vi "LDA_Beam_Alignment.vi"() -> ()   [LabVIEW 2021]
uses:
  Anemometry Sub Vis/Controls/Beam_Type.ctl
  Anemometry Sub Vis/Controls/Fixed Axis.ctl
  Anemometry Sub Vis/Gen Trav/Traverse_cluster.ctl
  Anemometry Sub Vis/Gen Trav/Spacing.ctl
  Anemometry Sub Vis/Controls/Multi_run_mode.ctl
  Anemometry Sub Vis/Controls/User_Specific_mode.ctl
  Anemometry Sub Vis/Controls/Tunnel_Coordinates.ctl
  Anemometry Sub Vis/Controls/Post_Process.ctl
  Anemometry Sub Vis/Gen Trav/Trav_mode.ctl
  Anemometry Sub Vis/Globals/Trav_pos_global.vi
  Anemometry Sub Vis/Globals/Meas_global.vi
panel:
  out "String":string
  in  "Peak up":bool[](array[boolean])
  out "Fixed Axis":T1
  out "Beam Names":string[](array[string])
  in  "Mode":T2(ring)
  out "Values Out":dbl[][](array[numeric])
  out "Message":string
  in  "Go Back":bool
  in  "OK":bool
  in  "stop":bool
  in  "Working On":T3 items=["532 Unshifted", "532 shifted", "561 Unshfited", "561 Shfited", "553 Unshfited", "553 Shfited"]
  # "X                 Y              Z           Power mW"
  # "X                 Y              Z"
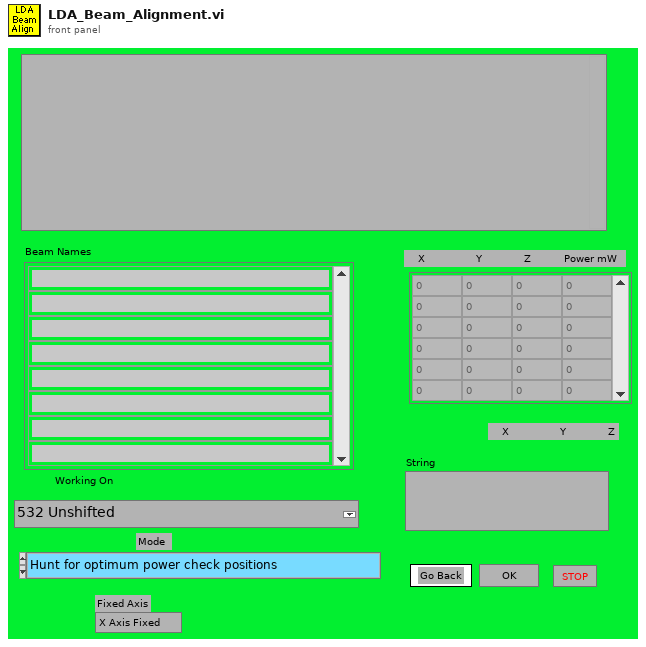
[diagram p1: front panel]
types:
  T1 = typedef "Fixed Axis.ctl" = enum16{"X Axis Fixed", "Y Axis Fixed", "Z Axis Fixed"}
  T2 = enum16{"Hunt for optimum power check positions", "Check Beam powers now", "Peak up beam power using manipulators"}
  T3 = typedef "Beam_Type.ctl" = u16
  T4 = typedef "Traverse_cluster.ctl" = cluster{"Start X":sgl, "Start Y":sgl, "Start Z":sgl, "End X":sgl, "End Y":sgl, "End Z":sgl, "nPoints":i32, "Spacing":T5, "Filename":path, "Tunnel Speed":dbl, "Averaging time (mins)":dbl, "Extra Commands":string, "Carrier_1 Q (l/min)":dbl, "Carrier_2 Q (l/min)":dbl, "Trace Gas Concentration (%)":dbl, "Specific Arguments":string, "Comments":string, "Row No":i32, "Row Type Selector":T6, "EstCompl":string, "Row Duration (mins)":dbl, "nValidPoints":i32, "Meas Setup File":string}
  T5 = typedef "Spacing.ctl" = enum16{"Linear", "Log", "Gauss", "Specified", "N/A"}
  T6 = typedef "Multi_run_mode.ctl" = enum16{"Move Traverse Only", "Set Tunnel Speed Only", "Set Source Only", "Set Measurement Conditions", "Single Measurement", "Vertical Profile", "Lateral Profile", "Longitudinal Profile", "Multi-Axis Profile", "Explore Volume", "Auto Calibrate", "Meas Fast FID Bkgnd", "Check Beam Power", "Scanning Valve Measurement", "Run VI Named:", "Set ADAM Ch", "Wait (minutes)", "Send Message", "Synchronize With:", "Fall Back to this Row", "Turn Off Row Repeating", "Traverse 3D Volume", "Blank Row", "Jump to Fall Back Row"}
  T7 = cluster{"Position":dbl[], "Traverse Name":string}[][]
  T8 = typedef "Tunnel_Coordinates.ctl" = enum16{"Work in Tunnel Coordinates", "Work in Model Coordinates"}
  T9 = typedef "User_Specific_mode.ctl" = enum16{"Check VI only", "Run VI"}
  T10 = typedef "Post_Process.ctl" = enum16{"Take New Data", "Post Process Raw Data File"}
  T11 = typedef "Trav_mode.ctl" = enum16{"Move traverse", "Read traverse position", "Teach Position"}
  T12 = cluster{"Position":dbl[], "Traverse Name":string}[]
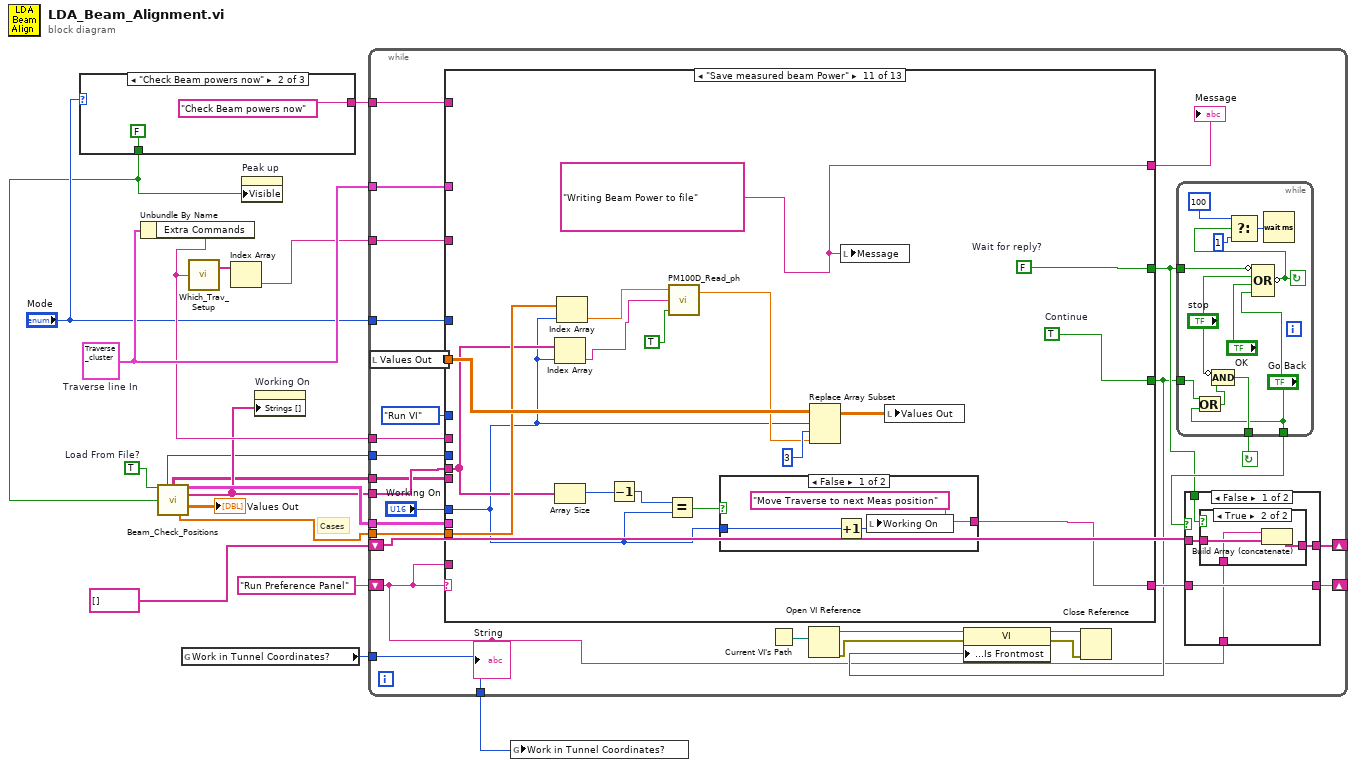
[diagram p0: block diagram]
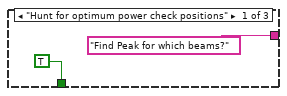
[diagram p2: hidden frame]
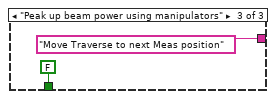
[diagram p3: hidden frame]
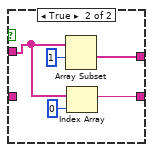
[diagram p5: hidden frame]
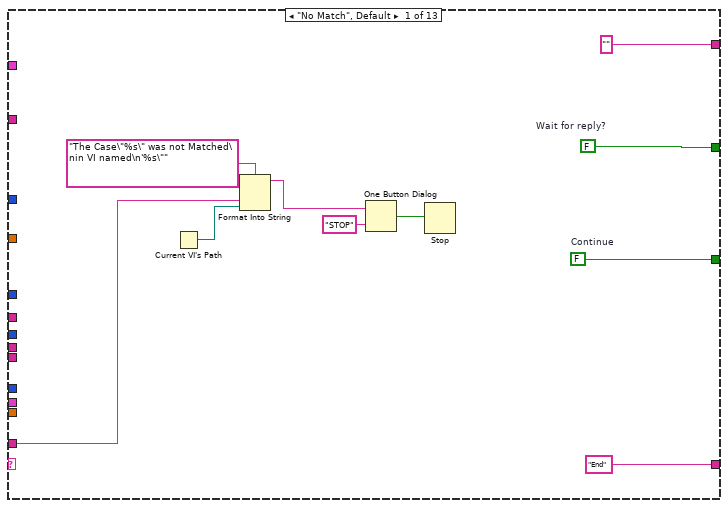
[diagram p6: hidden frame]
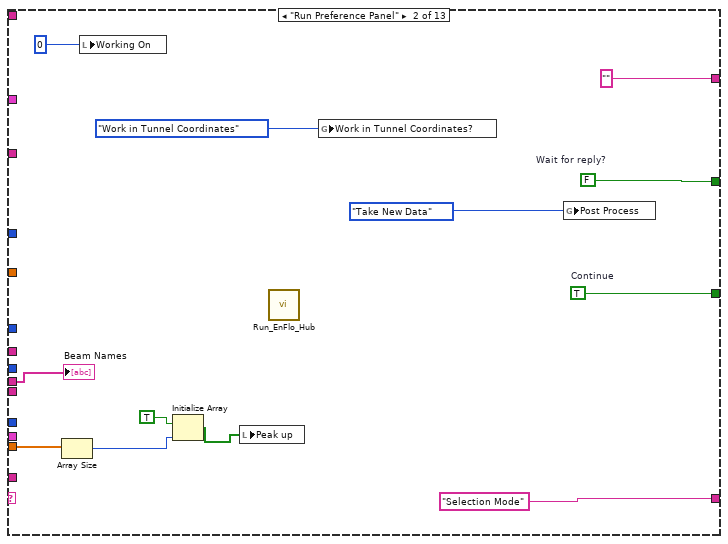
[diagram p7: hidden frame]
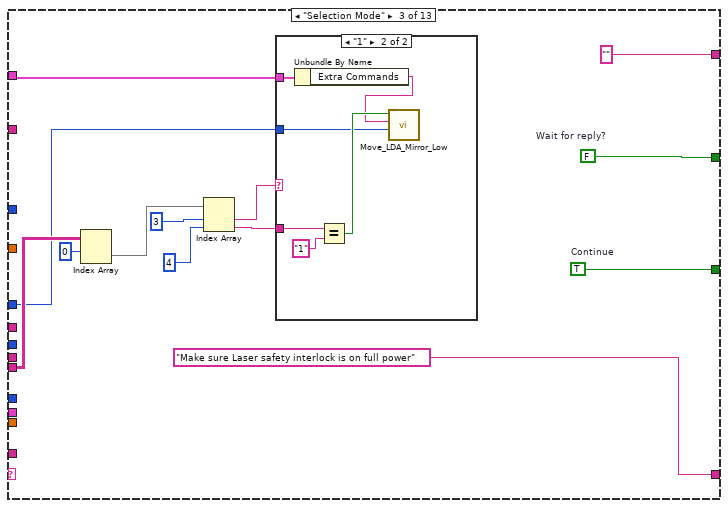
[diagram p8: hidden frame]
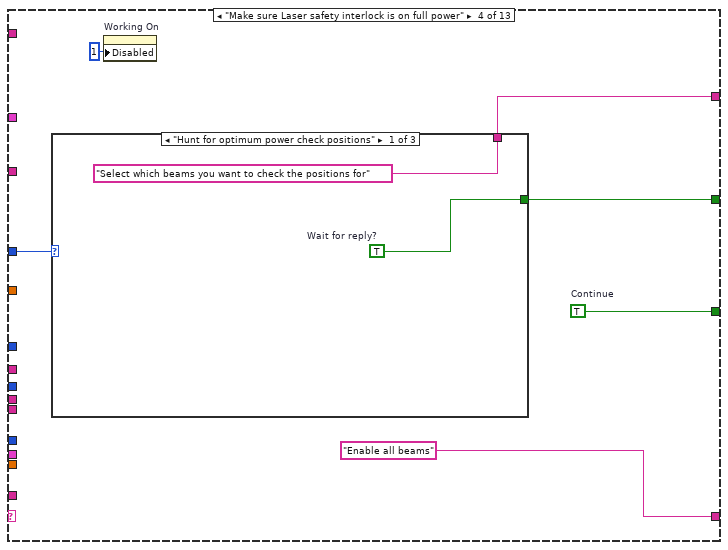
[diagram p10: hidden frame]
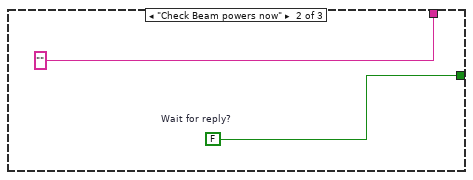
[diagram p11: hidden frame]
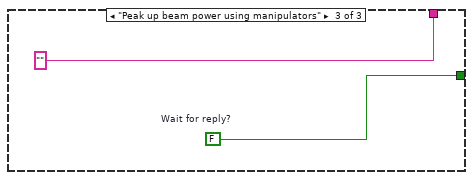
[diagram p12: hidden frame]
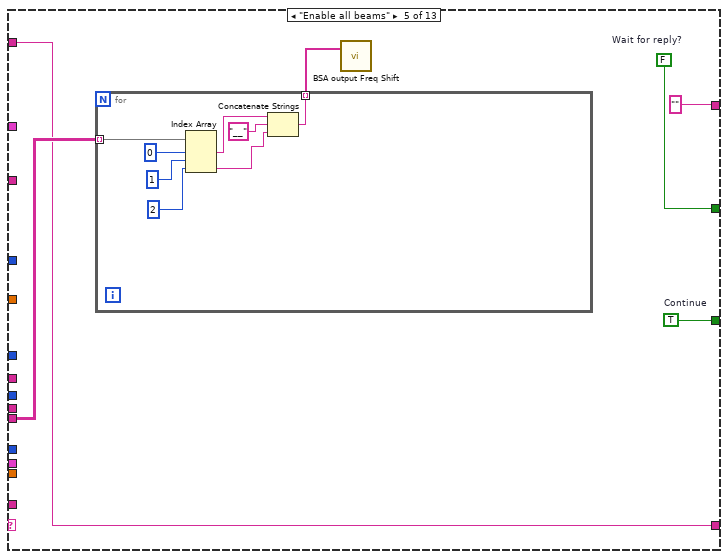
[diagram p13: hidden frame]
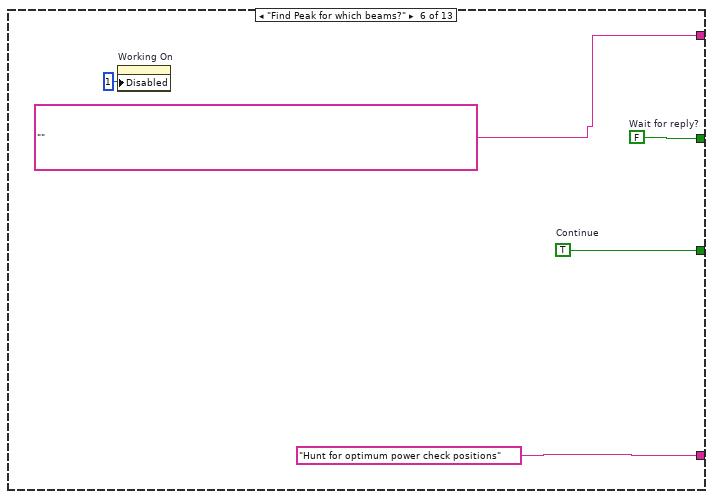
[diagram p14: hidden frame]
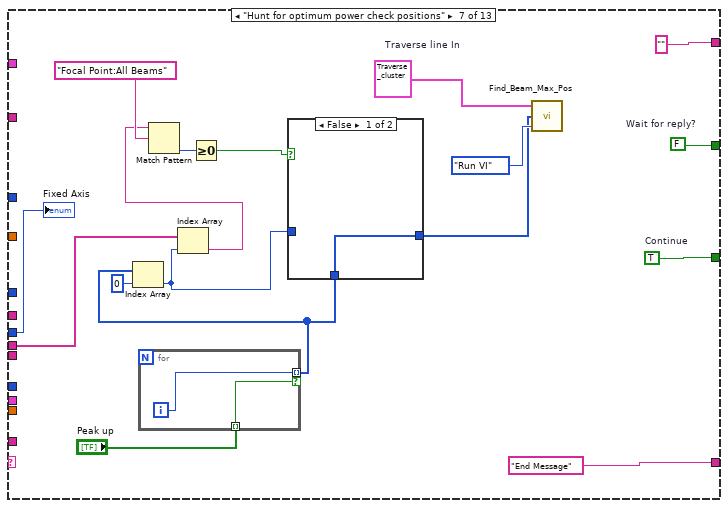
[diagram p15: hidden frame]
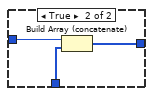
[diagram p16: hidden frame]
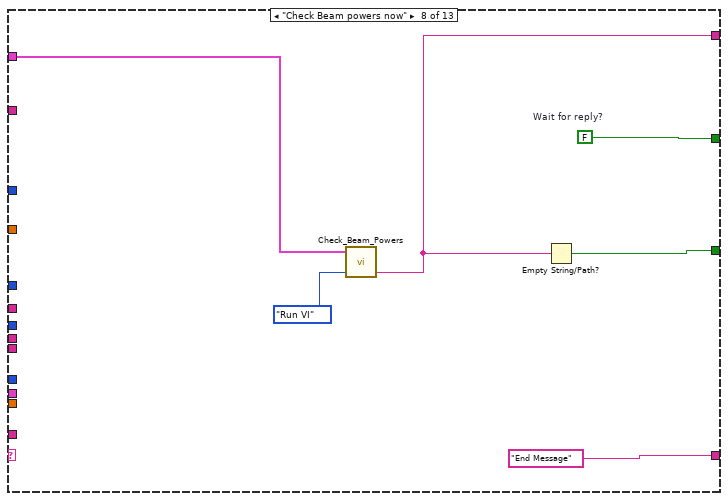
[diagram p17: hidden frame]
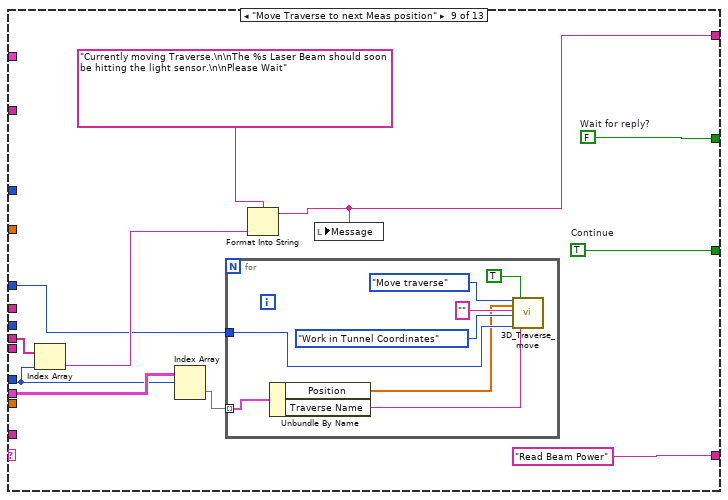
[diagram p18: hidden frame]
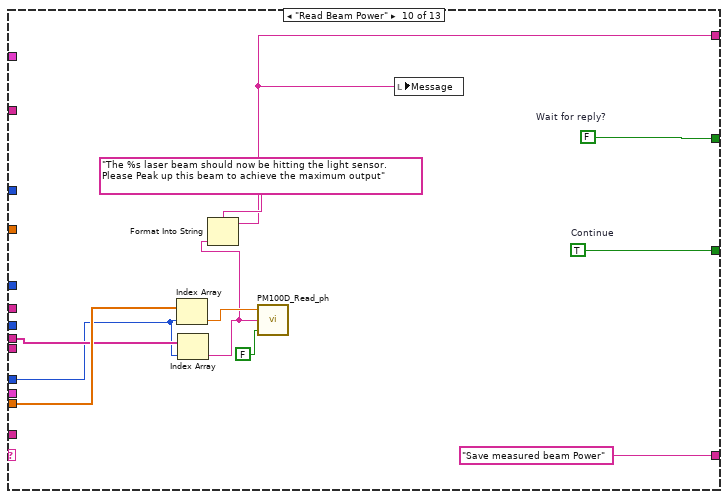
[diagram p19: hidden frame]
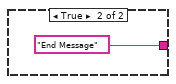
[diagram p20: hidden frame]
diagram:
  w10 = TRUE  # Load From File?
  w13 = T4 {"Start X"=0.0, "Start Y"=0.0, "Start Z"=0.0, "End X"=0.0, "End Y"=0.0, "End Z"=0.0, "nPoints"=0, "Spacing"=enum."Linear", "Filename"=path "", "Tunnel Speed"=0.0, "Averaging time (mins)"=0.0, "Extra Commands"="", "Carrier_1 Q (l/min)"=0.0, "Carrier_2 Q (l/min)"=0.0, "Trace Gas Concentration (%)"=0.0, "Specific Arguments"="", "Comments"="", "Row No"=0, "Row Type Selector"=enum."Move Traverse Only", "EstCompl"="", "Row Duration (mins)"=0.0, "nValidPoints"=0, "Meas Setup File"=""}  # Traverse line In
  # "Cases"
  n1 = case shown="\"Check Beam powers now\"" "Mode" {
    tunnel: ["Find Peak for which beams?" "Check Beam powers now" "Move Traverse to next Meas position"] -> w2
    tunnel: [TRUE FALSE FALSE] -> w1
    frame "Hunt for optimum power check positions" {
    }
    frame "Check Beam powers now" {
    }
    frame "Peak up beam power using manipulators" {
    }
  }
  n2 = Unbundle By Name(w13) -> ("Extra Commands"=w11:string)
  n3 = call "Beam_Check_Positions.vi"("Load From File?"=w10, "Give Focal Point Info (F)"=w1) -> ("Fixed Axis"=w5:T1, "More Info"=w4:string[][], "Beam Info"=w9:T7, "Beam Names"=w6:string[], "Primary Beam Positions"=→"Values Out":dbl[][], "Wavelength (nm)"=w7:dbl[])  [unwired: 5 in, 3 out]
  n4 = global read "Trav_pos_global.vi" "Work in Tunnel Coordinates?"() -> (w15:T8)
  n5 = call "Which_Trav_Setup.vi"("Extra Command String"=w11) -> ("Traverse Setups"=w14:string[])  [unwired: 2 out]
  n6 = Index Array(array=w14) -> (element=w12:string)  [unwired: 1 in]
  n7 = property on="Peak up" class="Arr (strict)"("Visible"=w1) -> ()  [unwired: 2 in, 2 out]
  n8 = property on="Working On" class="Ring (strict)"("Strings []"=w6) -> ()  [unwired: 2 in, 2 out]
  n9 = while {
    tunnel: w13 -> [w36]
    tunnel: "Mode" -> [w37]
    shift-left: string[] [] -> [w51]
    shift-right: [w50] -> _
    shift-left: "Run Preference Panel" -> [w35]
    shift-right: [w49] -> _
    tunnel: [w34] -> w16
    tunnel: w15 -> [w34]
    tunnel: w12 -> [w33]
    tunnel: w11 -> [w32]
    tunnel: w9 -> [w31]
    tunnel: w6 -> [w29]
    tunnel: w7 -> [w28]
    tunnel: w5 -> [w27]
    tunnel: w4 -> [w26]
    tunnel: w2 -> [w25]
    stop <- w53 continue-if-true
    n10 = local read "Values Out"() -> (w38:dbl[][])
    n11 = case shown="\"Save measured beam Power\"" w35 {
      tunnel: [w88 w100 w113 w125 w137 w150 w164 w174 w190 w209 w226 w234 w248] -> w40
      tunnel: ["End" "Selection Mode" "Make sure Laser safety interlock is on full power" "Enable all beams" w132 "Hunt for optimum power check positions" "End Message" "End Message" "Read Beam Power" "Save measured beam Power" w220 "End Message" "End"] -> w48
      tunnel: [w87 w99 w112 w120 w136 w149 w165 w177 w189 w208 w225 w233 w247] -> w41
      tunnel: ["" "" "" w121 "" "" "" w175 w180 w199 w219 "Now open all the individual shutters so all four beam are showing." w241] -> w30
      tunnel: User_Specific_mode."Run VI" ("Simulate/Run") -> [_ _ w101 _ _ _ _ _ w182 _ _ _ _]
      tunnel: w29 -> [_ w90 _ _ _ _ w156 _ w187 w203 w213 _ w237]
      tunnel: "Working On" -> [_ _ _ _ _ _ _ _ w181 w202 w212 _ _]
      tunnel: w38 -> [_ _ _ _ _ _ _ _ _ _ w223 _ _]
      tunnel: w37 -> [_ _ _ w122 _ _ _ _ _ _ _ _ w244]
      tunnel: w36 -> [_ _ w103 _ _ _ _ w176 _ _ _ _ _]
      tunnel: w35 -> [w79 _ _ _ _ _ _ _ _ _ _ _ _]
      tunnel: w33 -> [_ _ _ _ _ _ _ _ _ _ _ _ _]
      tunnel: w32 -> [_ _ _ _ _ _ _ _ _ _ _ _ _]
      tunnel: w31 -> [_ _ _ _ _ _ _ _ w183 _ _ _ _]
      tunnel: w28 -> [_ w94 _ _ _ _ _ _ _ w204 w217 _ _]
      tunnel: w27 -> [_ _ _ _ _ _ w161 _ _ _ _ _ _]
      tunnel: w26 -> [_ _ w102 _ w134 _ _ _ _ _ _ _ _]
      tunnel: w25 -> [_ _ _ _ w132 _ _ _ _ _ _ _ _]
      frame "No Match", Default {
        w87 = FALSE  # Wait for reply?
        w88 = FALSE  # Continue
        n12 = Current VI's Path() -> (path=w80:path)
        n13 = Format Into String(format string="The Case\"%s\" was not Matched\nin VI named\n'%s\"" ("Format String"), w79, w80) -> (resulting string=w83:string)  [unwired: 2 in, 1 out]
        n14 = One Button Dialog(message=w83, button name ("OK")="STOP") -> (true=w81:bool)
        n15 = Stop(stop? (T)=w81) -> ()
      }
      frame "Run Preference Panel" {
        w99 = FALSE  # Wait for reply?
        w100 = TRUE  # Continue
        n16 = Array Size(array=w94) -> (size(s)=w93:i32)
        n17 = local write "Working On"(0) -> ()
        n18 = Initialize Array(TRUE, w93) -> (w91:bool[])
        n19 = local write "Peak up"(w91) -> ()
        n20 = call "Run_EnFlo_Hub.vi"() -> ()  [unwired: 1 in, 7 out]
        n21 = global write "Trav_pos_global.vi" "Work in Tunnel Coordinates?"(Tunnel_Coordinates."Work in Tunnel Coordinates" ("Work in Tunnel Coordinates?")) -> ()
        n22 = global write "Meas_global.vi" "Post Process"(Post_Process."Take New Data" ("Post Process")) -> ()
        "Beam Names" <- w90
      }
      frame "Selection Mode" {
        w112 = FALSE  # Wait for reply?
        w113 = TRUE  # Continue
        n23 = Index Array(array=w102, index (row)=0) -> (element=w105:string[])  [unwired: 1 in]
        n24 = Index Array(array=w105, index #1=3 ("index"), index #2=4 ("index")) -> (element #1=w108:string, element #2=w109:string)
        n25 = case shown="\"1\"" w108 {
          tunnel: w101 -> [_ w114]
          tunnel: w109 -> [_ w119]
          tunnel: w103 -> [_ w116]
          frame Default {
          }
          frame "1" {
            n26 = Unbundle By Name(w116) -> ("Extra Commands"=w115:string)
            n27 = Equal?(x=w119, y="1") -> (x = y?=w117:bool)
            n28 = call "Move_LDA_Mirror_Low.vi"("Mode"=w114, "Extra Commands"=w115, "Mirror Up?"=w117) -> ()  [unwired: 1 in, 2 out]
          }
        }
      }
      frame "Make sure Laser safety interlock is on full power" {
        w125 = TRUE  # Continue
        n29 = case shown="\"Hunt for optimum power check positions\"" w122 {
          tunnel: ["Select which beams you want to check the positions for" "" ""] -> w121
          tunnel: [w126 w128 w130] -> w120
          frame "Hunt for optimum power check positions" {
            w126 = TRUE  # Wait for reply?
          }
          frame "Check Beam powers now" {
            w128 = FALSE  # Wait for reply?
          }
          frame "Peak up beam power using manipulators" {
            w130 = FALSE  # Wait for reply?
          }
        }
        n30 = property on="Working On" class="Ring (strict)"("Disabled"=u8 1 ("Write Attribute")) -> ()  [unwired: 2 in, 2 out]
      }
      frame "Enable all beams" {
        w136 = FALSE  # Wait for reply?
        w137 = TRUE  # Continue
        n31 = for {
          tunnel: w134 -> [w142] mode=indexing
          tunnel: [w139] -> w133 mode=indexing
          n32 = Index Array(array=w142, index #1=0 ("index"), index #2=1 ("index"), index #3=2 ("index")) -> (element #1=w141:string, element #3=w140:string)  [unwired: 1 out]
          n33 = Concatenate Strings(w141, "__" ("string"), w140) -> (w139:string)
        }
        n34 = call "BSA output Freq Shift.vi"("BSAIP__ChNum"=w133) -> ()  [unwired: 2 in, 1 out]
      }
      frame "Find Peak for which beams?" {
        w149 = FALSE  # Wait for reply?
        w150 = TRUE  # Continue
        n35 = property on="Working On" class="Ring (strict)"("Disabled"=u8 1 ("Write Attribute")) -> ()  [unwired: 2 in, 2 out]
      }
      frame "Hunt for optimum power check positions" {
        w165 = FALSE  # Wait for reply?
        w164 = TRUE  # Continue
        w162 = T4 {"Start X"=0.0, "Start Y"=0.0, "Start Z"=0.0, "End X"=0.0, "End Y"=0.0, "End Z"=0.0, "nPoints"=0, "Spacing"=enum."Linear", "Filename"=path "", "Tunnel Speed"=0.0, "Averaging time (mins)"=0.0, "Extra Commands"="", "Carrier_1 Q (l/min)"=0.0, "Carrier_2 Q (l/min)"=0.0, "Trace Gas Concentration (%)"=0.0, "Specific Arguments"="", "Comments"="", "Row No"=0, "Row Type Selector"=enum."Move Traverse Only", "EstCompl"="", "Row Duration (mins)"=0.0, "nValidPoints"=0, "Meas Setup File"=""}  # Traverse line In
        n36 = for {
          tunnel: [w173] -> w153 mode=indexing if=w172
          tunnel: "Peak up" -> [w172] mode=indexing
          i -> [w173]
        }
        n37 = Index Array(array=w153, index=0) -> (element=w152:i32)
        n38 = Index Array(array=w156, index=w152) -> (element=w155:string)
        n39 = Match Pattern(string=w155, regular expression="Focal Point:All Beams") -> (offset past match=w157:i32)  [unwired: 1 in, 3 out]
        n40 = Greater Or Equal To 0?(x=w157) -> (x >= 0?=w154:bool)
        n41 = case shown="False" w154 {
          tunnel: w153 -> [w168 w171]
          tunnel: w152 -> [_ w170]
          tunnel: [w168 w169] -> w151
          frame False {
          }
          frame True {
            n42 = Build Array (concatenate)(w170, w171) -> (w169:i32[])
          }
        }
        n43 = call "Find_Beam_Max_Pos.vi"("Mode"=User_Specific_mode."Run VI", "Beams to peak up"=w151, "Traverse line In"=w162) -> ()  [unwired: 3 out]
        "Fixed Axis" <- w161
      }
      frame "Check Beam powers now" {
        w177 = FALSE  # Wait for reply?
        n44 = call "Check_Beam_Powers.vi"("Mode"=User_Specific_mode."Run VI", "Traverse line In"=w176) -> ("Error Message"=w175:string)  [unwired: 1 in, 2 out]
        n45 = Empty String/Path?(string/path=w175) -> (empty?=w174:bool)
      }
      frame "Move Traverse to next Meas position" {
        w189 = FALSE  # Wait for reply?
        w190 = TRUE  # Continue
        n46 = Index Array(array=w187, index=w181) -> (element=w185:string)
        n47 = Index Array(array=w183, index (row)=w181) -> (element=w184:T12)  [unwired: 1 in]
        n48 = for {
          tunnel: w184 -> [w193] mode=indexing
          tunnel: w182 -> [w194]
          n49 = Unbundle By Name(w193) -> ("Position"=w192:dbl[], "Traverse Name"=w191:string)
          n50 = call "3D_Traverse_move.vi"("Mode"=Trav_mode."Move traverse", "Position"=w192, "Extra command String"="", "Work in Tunnel Coordinates"=Tunnel_Coordinates."Work in Tunnel Coordinates", "Simulate/Run"=w194, "Route Checking?"=TRUE, "Traverse name"=w191) -> ()  [unwired: 9 in, 4 out]
        }
        n51 = Format Into String(format string="Currently moving Traverse.\n\nThe %s Laser Beam should soon be hitting the light sensor.\n\nPlease Wait", w185) -> (resulting string=w180:string)  [unwired: 2 in, 1 out]
        n52 = local write "Message"(w180) -> ()
      }
      frame "Read Beam Power" {
        w208 = FALSE  # Wait for reply?
        w209 = TRUE  # Continue
        n53 = Index Array(array=w204, index=w202) -> (element=w206:dbl)
        n54 = Index Array(array=w203, index=w202) -> (element=w200:string)
        n55 = Format Into String(format string="The %s laser beam should now be hitting the light sensor. Please Peak up this beam to achieve the maximum output", w200) -> (resulting string=w199:string)  [unwired: 2 in, 1 out]
        n56 = call "PM100D_Read_ph.vi"("stop"=FALSE, "Beam Name"=w200, "Wavelength (0.0)"=w206) -> ()  [unwired: 2 out]
        n57 = local write "Message"(w199) -> ()
      }
      frame "Save measured beam Power" {
        w219 = "Writing Beam Power to file"
        w225 = FALSE  # Wait for reply?
        w226 = TRUE  # Continue
        n58 = Index Array(array=w213, index=w212) -> (element=w214:string)
        n59 = Array Size(array=w213) -> (size(s)=w211:i32)
        n60 = Index Array(array=w217, index=w212) -> (element=w216:dbl)
        n61 = Decrement(x=w211) -> (x-1=w210:i32)
        n62 = Equal?(x=w210, y=w212) -> (x = y?=w221:bool)
        n63 = call "PM100D_Read_ph.vi"("stop"=TRUE, "Beam Name"=w214, "Wavelength (0.0)"=w216) -> ("Average Power (mW)"=w215:dbl)  [unwired: 1 out]
        n64 = case shown="False" w221 {
          tunnel: ["Move Traverse to next Meas position" "End Message"] -> w220
          tunnel: w212 -> [w229 _]
          frame False {
            n65 = Increment(x=w229) -> (x+1=w228:T3)
            n66 = local write "Working On"(w228) -> ()
          }
          frame True {
          }
        }
        n67 = Replace Array Subset(array=w223, new element=w215, index (row)=w212, index (col)=3 ("Index")) -> (w222:dbl[][])
        n68 = local write "Message"(w219) -> ()
        n69 = local write "Values Out"(w222) -> ()
      }
      frame "Open all individual laser shutters again" {
        w233 = TRUE  # Wait for reply?
        w234 = TRUE  # Continue
      }
      frame "End Message" {
        w239 = TRUE  # Load From File?
        w247 = FALSE  # Wait for reply?
        w248 = FALSE  # Continue
        n70 = property on="Mode" class="Enum (strict)"() -> ("Strings []"=w245:string[])  [unwired: 2 in, 2 out]
        n71 = Index Array(array=w237) -> (element=w236:string)  [unwired: 1 in]
        n72 = Index Array(array=w245, index=w244) -> (element=w243:string)
        n73 = Equal?(x="Focal Point:All Beams" ("regular expression"), y=w236) -> (x = y?=w235:bool)
        n74 = Format Into String(format string="%s\nhas now been completed" ("Format String"), w243) -> (resulting string=w241:string)  [unwired: 2 in, 1 out]
        n75 = case shown="True" w235 {
          frame False {
          }
          frame True {
            n76 = call "Update Beam Separations.vi"() -> ()  [unwired: 12 in]
          }
        }
        n77 = call "Beam_Check_Positions.vi"("Load From File?"=w239) -> ("Primary Beam Positions"=w240:dbl[][])  [unwired: 6 in, 8 out]
        n78 = local write "Values Out"(w240) -> ()
      }
    }
    "Message" <- w30
    n79 = Current VI's Path() -> (path=w46:path)
    n80 = Open VI Reference(vi path=w46) -> (vi reference=w45:refnum<vi>, error out=w44:errorcluster)  [unwired: 1 in, 4 out]
    n81 = property class="VI"(reference=w45, error in=w44, "Front Panel Window:Is Frontmost"=w40) -> (reference out=w43:refnum<vi>, error out=w42:errorcluster)
    n82 = Close Reference(reference=w43, error in (no error)=w42) -> ()  [unwired: 1 out]
    n83 = while {
      tunnel: ["Go Back"] -> w52
      tunnel: [w61] -> w53
      tunnel: w40 -> [w60]
      tunnel: w41 -> [w63]
      stop <- w57 continue-if-true
      n84 = Or(x=w60, y="Go Back") -> (x .or. y?=w58:bool)
      n85 = Compound Arithmetic op=AND(invert "stop", w58) -> (w61:bool)
      n86 = Compound Arithmetic op=OR(invert w63, "stop", "OK", "Go Back") -> (invert w57:bool)
      n87 = Select(t=u32 100 ("millisecond timer value"), s=w57, f=u32 1) -> (s? t:f=w54:u32)
      n88 = Wait (ms)(milliseconds to wait=w54) -> ()  [unwired: 1 out]
    }
    n89 = case shown="False" w52 {
      tunnel: w51 -> [w69 w74]
      tunnel: [w68 w75] -> w50
      tunnel: w35 -> [w66 _]
      tunnel: [w67 w76] -> w49
      tunnel: w48 -> [w67 _]
      tunnel: w41 -> [w65 _]
      frame False {
        n90 = case shown="True" w65 {
          tunnel: w69 -> [w70 w73]
          tunnel: [w70 w72] -> w68
          tunnel: w66 -> [_ w71]
          frame False {
          }
          frame True {
            n91 = Build Array (concatenate)(w71, w73) -> (w72:string[])
          }
        }
      }
      frame True {
        n92 = Array Subset(array=w74, index=1 ("Array Index")) -> (w75:string[])  [unwired: 1 in]
        n93 = Index Array(array=w74, index=0 ("Index")) -> (element=w76:string)
      }
    }
    "String" <- w35
  }
  n94 = global write "Trav_pos_global.vi" "Work in Tunnel Coordinates?"(w16) -> ()
